vi "MBK System simulation.vi"() -> ()   [LabVIEW 2018]
uses:
  <vilib>/Analysis/3filter.llb/Filter Passband Type.ctl
  <vilib>/DAQmx/write.llb/DAQmx Write (Analog 1D DBL NChan 1Samp).vi
  <vilib>/DAQmx/read.llb/DAQmx Read (Analog 1D DBL NChan 1Samp).vi
  <vilib>/DAQmx/create/channels.llb/DAQmx Create Channel (AO-Voltage-Basic).vi
  <vilib>/DAQmx/create/channels.llb/DAQmx Create Channel (AI-Voltage-Basic).vi
  <vilib>/DAQmx/miscellaneous.llb/DAQmx Fill In Error Info.vi
  <vilib>/ptbypt/NI_PtbyPt.lvlib
  <vilib>/Analysis/NI_AALBase.lvlib
panel:
  out "Measured Acceleration":dbl(graph)
  in  "K":dbl min=0.0 max=10.0 step=0.001
  in  "Force filter Y/N":bool
  out "Desired Vel":dbl(graph)
  out "Desired acc":dbl(graph)
  in  "I_app_wall":dbl min=0.0 max=1.0 step=1e-05
  in  "I_app_transp":dbl=1e-06 min=1e-06 max=0.1 step=1e-06
  in  "B":dbl min=0.0 max=1.0 step=0.0001
  out "Velocity Meas":dbl(graph)
  in  "Vel Fil Y/N":bool
  in  "Loop Frequency":dbl
  out "Position Measured":dbl(graph)
  in  "Pos Fil Y/N":bool
  out "Force measure":dbl(graph)
  in  "stop":bool
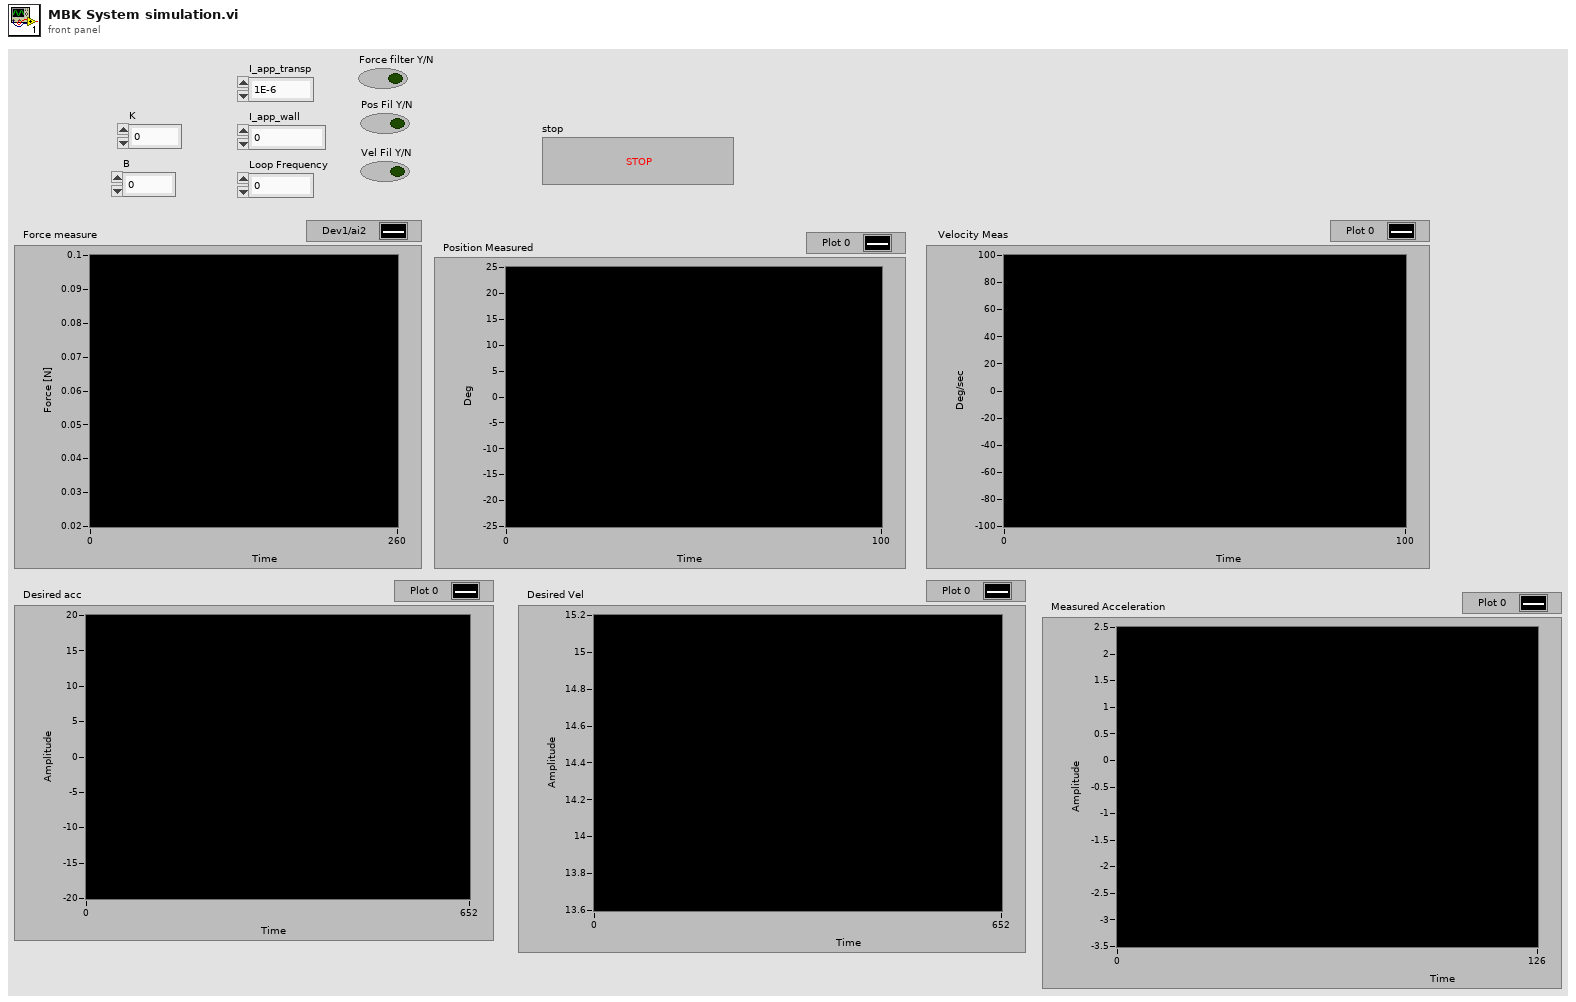
[diagram p1: front panel]
types:
  T1 = typedef "NI_AALBase.lvlib/Filter Passband Type.ctl" = enum32{"Lowpass", "Highpass", "Bandpass", "Bandstop"}
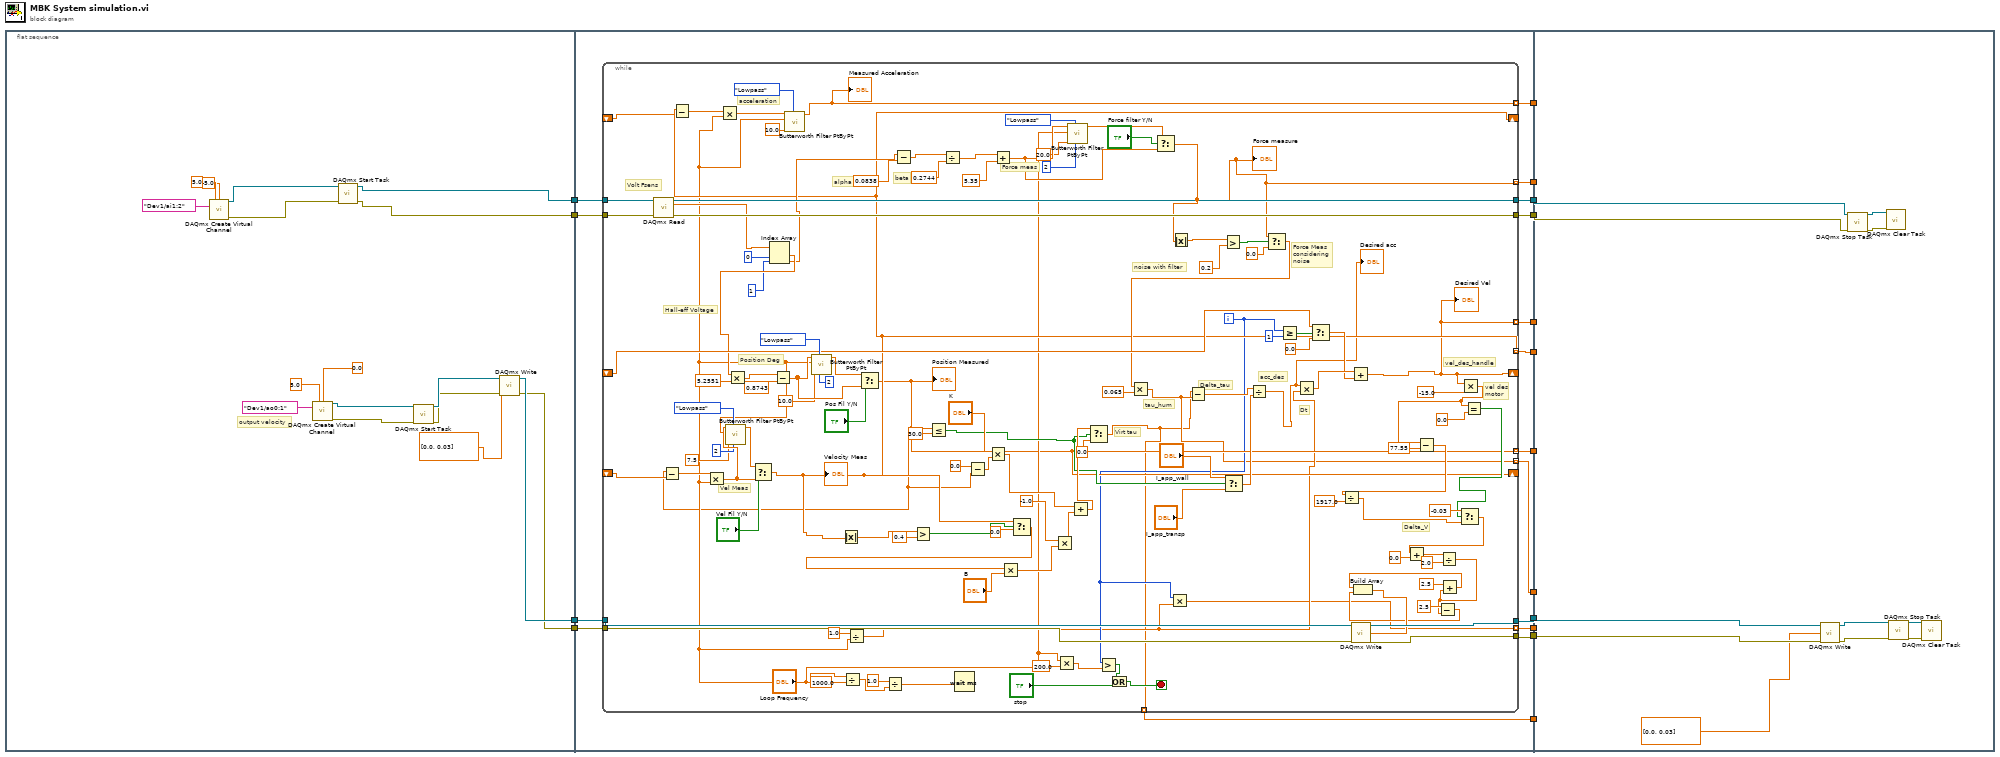
[diagram p0: block diagram]
diagram:
  n1 = flat-sequence {
    tunnel: [w30] -> w14
    tunnel: [w27] -> w12
    tunnel: [w17] -> w10
    tunnel: [w18] -> w9
    tunnel: [w49] -> w16
    tunnel: [w48] -> w15
    tunnel: w14 -> [w47]
    tunnel: [w46] -> w13
    tunnel: w12 -> [w45]
    tunnel: [w44] -> w11
    tunnel: w10 -> [w43]
    tunnel: w9 -> [w42]
    tunnel: [w41] -> w8
    tunnel: [w40] -> w7
    tunnel: [w39] -> w6
    tunnel: [w38] -> w5
    tunnel: [w37] -> w4
    tunnel: [w36] -> w3
    tunnel: [w35] -> w2
    tunnel: [w34] -> w1
    tunnel: w16 -> [w180]
    tunnel: w15 -> [w178]
    tunnel: w13 -> [w174]
    tunnel: w11 -> [w172]
    tunnel: w8 -> [_]
    tunnel: w7 -> [_]
    tunnel: w6 -> [_]
    tunnel: w5 -> [_]
    tunnel: w4 -> [_]
    tunnel: w3 -> [_]
    tunnel: w2 -> [_]
    tunnel: w1 -> [_]
    frame #0 {
      # "output velocity"
      n2 = call-poly <vilib>:"DAQmx Create Virtual Channel.vi"("maximum value"=5.0, "minimum value"=-5.0, "physical channels"=tag "Dev1/ai1:2") -> ("task out"=w24:refnum<k21>, "error out"=w23:errorcluster)  [unwired: 11 in]
      n3 = call-poly <vilib>:"DAQmx Create Virtual Channel.vi"("maximum value"=5.0, "minimum value"=0.0, "physical channels"=tag "Dev1/ao0:1") -> ("task out"=w32:refnum<k21>, "error out"=w29:errorcluster)  [unwired: 11 in]
      n4 = call <vilib>:"DAQmx Start Task.vi"("task/channels in"=w24, "error in"=w23) -> ("task out"=w18:refnum<k21>, "error out"=w17:errorcluster)  [unwired: 12 in]
      n5 = call <vilib>:"DAQmx Start Task.vi"("task/channels in"=w32, "error in"=w29) -> ("task out"=w31:refnum<k21>, "error out"=w28:errorcluster)  [unwired: 12 in]
      n6 = call-poly <vilib>:"DAQmx Write.vi"("task/channels in"=w31, "data"=dbl[] [0.0, 0.03], "error in"=w28) -> ("task out"=w30:refnum<k21>, "error out"=w27:errorcluster)  [unwired: 10 in, 1 out]
    }
    frame #1 {
      n7 = while {
        tunnel: [w169] -> w49
        tunnel: [w168] -> w48
        tunnel: w47 -> [w164]
        tunnel: [w163] -> w46
        tunnel: w45 -> [w162]
        tunnel: [w161] -> w44
        shift-right: [w59] -> _
        shift-left: _ -> [w99]
        tunnel: w43 -> [w137]
        tunnel: w42 -> [w136]
        shift-right: [w52] -> _
        shift-left: _ -> [w122]
        tunnel: [w75] -> w41 mode=indexing
        tunnel: [w74] -> w40 mode=indexing
        shift-right: [w74] -> _
        shift-left: _ -> [w73]
        tunnel: [w62] -> w39 mode=indexing
        tunnel: [w52] -> w38 mode=indexing
        tunnel: [w59] -> w37 mode=indexing
        tunnel: [w51] -> w36 mode=indexing
        tunnel: [w50] -> w35 mode=indexing
        tunnel: [w56] -> w34 mode=indexing
        i -> [w58]
        stop <- w63 stop-if-true
        # "acceleration"
        # "vel des\nmotor"
        # "Dt"
        # "Force Meas\nconsidering\nnoise"
        # "noise with filter"
        # "Force meas"
        # "Virt tau"
        # "Vel Meas"
        # "Hall-eff Voltage"
        # "Delta_tau"
        # "tau_hum"
        # "vel_des_handle"
        # "Delta_V"
        # "acc_des"
        # "Position Deg"
        # "Volt Fsens"
        # "beta"
        # "alpha"
        n8 = call-poly <vilib>:"DAQmx Read.vi"("task/channels in"=w136, "error in"=w137) -> ("task out"=w169:refnum<k21>, "data"=w138:dbl[], "error out"=w168:errorcluster)  [unwired: 11 in]
        n9 = Index Array(array=w138, index #1=0 ("index"), index #2=1 ("index")) -> (element #1=w107:dbl, element #2=w106:dbl)
        n10 = Multiply(x=w107, y=5.2551) -> (x*y=w159:dbl)
        n11 = Subtract(x=w159, y=0.8743) -> (x-y=w155:dbl)
        n12 = call <vilib>:"Butterworth Filter PtByPt.vi"("order"=2, "filter type"=Filter_Passband_Type."Lowpass", "low cutoff freq: fl"=10.0, "sampling freq: fs"="Loop Frequency", "x"=w155) -> ("Filtered x"=w156:dbl)  [unwired: 4 in, 1 out]
        n13 = Divide(x="Loop Frequency", y=1000.0) -> (x/y=w150:dbl)
        n14 = Divide(x=1.0, y="Loop Frequency") -> (x/y=w57:dbl)
        n15 = Select(t=w156, s="Pos Fil Y/N", f=w155) -> (s? t:f=w59:dbl)
        "Position Measured" <- w59
        n16 = Subtract(x=w59, y=w99) -> (x-y=w147:dbl)
        n17 = Multiply(x=w147, y="Loop Frequency") -> (x*y=w145:dbl)
        n18 = call <vilib>:"Butterworth Filter PtByPt.vi"("order"=2, "filter type"=Filter_Passband_Type."Lowpass", "low cutoff freq: fl"=7.5, "sampling freq: fs"="Loop Frequency", "x"=w145) -> ("Filtered x"=w144:dbl)  [unwired: 4 in, 1 out]
        n19 = Select(t=w144, s="Vel Fil Y/N", f=w145) -> (s? t:f=w74:dbl)
        "Velocity Meas" <- w74
        n20 = Subtract(x=w74, y=w73) -> (x-y=w72:dbl)
        n21 = Multiply(x=w72, y="Loop Frequency") -> (x*y=w71:dbl)
        n22 = call <vilib>:"Butterworth Filter PtByPt.vi"("filter type"=Filter_Passband_Type."Lowpass", "low cutoff freq: fl"=10.0, "sampling freq: fs"="Loop Frequency", "x"=w71) -> ("Filtered x"=w62:dbl)  [unwired: 5 in, 1 out]
        "Measured Acceleration" <- w62
        n23 = Absolute Value(x=w74) -> (abs(x)=w98:dbl)
        n24 = Divide(x=1.0, y=w150) -> (x/y=w135:dbl)
        n25 = Subtract(x=w106, y=0.0838) -> (x-y=w167:dbl)
        n26 = Greater?(x=w98, y=0.4) -> (0:w96:bool)
        n27 = Less Or Equal?(x=w59, y=30.0) -> (x <= y?=w77:bool)
        n28 = Divide(x=w167, y=0.2744) -> (x/y=w118:dbl)
        n29 = Wait (ms)(milliseconds to wait=w135) -> ()  [unwired: 1 out]
        n30 = Subtract(x=0.0, y=w59) -> (x-y=w88:dbl)
        n31 = Multiply(x="K", y=w88) -> (x*y=w86:dbl)
        n32 = Add(x=w118, y=5.35) -> (x+y=w116:dbl)
        n33 = Select(t=w74, s=w96, f=0.0) -> (s? t:f=w94:dbl)
        n34 = Multiply(x=w94, y="B") -> (x*y=w102:dbl)
        n35 = Multiply(x=-1.0, y=w102) -> (x*y=w90:dbl)
        n36 = Multiply(x="Loop Frequency", y=200.0) -> (x*y=w66:dbl)
        n37 = call <vilib>:"Butterworth Filter PtByPt.vi"("order"=2, "filter type"=Filter_Passband_Type."Lowpass", "low cutoff freq: fl"=20.0, "sampling freq: fs"="Loop Frequency", "x"=w116) -> ("Filtered x"=w117:dbl)  [unwired: 4 in, 1 out]
        n38 = Add(x=w86, y=w90) -> (x+y=w85:dbl)
        n39 = Select(t=w85, s=w77, f=0.0) -> (s? t:f=w50:dbl)
        n40 = Greater?(x=w58, y=w66) -> (0:w65:bool)
        n41 = Or(x=w65, y="stop") -> (x .or. y?=w63:bool)
        n42 = Select(t=w117, s="Force filter Y/N", f=w116) -> (s? t:f=w75:dbl)
        "Force measure" <- w75
        n43 = Multiply(x=w58, y=w57) -> (x*y=w56:dbl)
        n44 = Absolute Value(x=w75) -> (abs(x)=w108:dbl)
        n45 = Greater?(x=w108, y=0.2) -> (0:w60:bool)
        n46 = Select(t="I_app_wall", s=w77, f="I_app_transp") -> (s? t:f=w61:dbl)
        n47 = Select(t=w75, s=w60, f=0.0) -> (s? t:f=w109:dbl)
        n48 = Multiply(x=w109, y=0.065) -> (x*y=w51:dbl)
        n49 = Subtract(x=w50, y=w51) -> (x-y=w103:dbl)
        n50 = Divide(x=w103, y=w61) -> (x/y=w53:dbl)
        "Desired acc" <- w53
        n51 = Greater Or Equal?(x=w58, y=1) -> (x >= y?=w124:bool)
        n52 = Multiply(x=w53, y=w57) -> (x*y=w125:dbl)
        n53 = Select(t=w122, s=w124, f=0.0) -> (s? t:f=w120:dbl)
        n54 = Add(x=w125, y=w120) -> (x+y=w52:dbl)
        "Desired Vel" <- w52
        n55 = Multiply(x=w52, y=-15.0) -> (x*y=w78:dbl)
        n56 = Subtract(x=w78, y=77.55) -> (x-y=w92:dbl)
        n57 = Divide(x=w92, y=1917.0) -> (x/y=w54:dbl)
        n58 = Equal?(x=w78, y=0.0) -> (x = y?=w76:bool)
        n59 = Select(t=-0.03, s=w76, f=w54) -> (s? t:f=w55:dbl)
        n60 = Add(x=w55, y=0.0) -> (x+y=w132:dbl)
        n61 = Divide(x=w132, y=2.0) -> (x/y=w128:dbl)
        n62 = Subtract(x=2.5, y=w128) -> (x-y=w82:dbl)
        n63 = Add(x=2.5, y=w128) -> (x+y=w83:dbl)
        n64 = Build Array(w83, w82) -> (w95:dbl[])
        n65 = call-poly <vilib>:"DAQmx Write.vi"("task/channels in"=w164, "data"=w95, "error in"=w162) -> ("task out"=w163:refnum<k21>, "error out"=w161:errorcluster)  [unwired: 10 in, 1 out]
      }
    }
    frame #2 {
      n66 = call-poly <vilib>:"DAQmx Write.vi"("task/channels in"=w174, "data"=dbl[] [0.0, 0.03], "error in"=w172) -> ("task out"=w173:refnum<k21>, "error out"=w171:errorcluster)  [unwired: 10 in, 1 out]
      n67 = call <vilib>:"DAQmx Stop Task.vi"("task/channels in"=w180, "error in"=w178) -> ("task out"=w179:refnum<k21>, "error out"=w177:errorcluster)  [unwired: 12 in]
      n68 = call <vilib>:"DAQmx Clear Task.vi"("task in"=w179, "error in"=w177) -> ()  [unwired: 13 in, 1 out]
      n69 = call <vilib>:"DAQmx Stop Task.vi"("task/channels in"=w173, "error in"=w171) -> ("task out"=w176:refnum<k21>, "error out"=w175:errorcluster)  [unwired: 12 in]
      n70 = call <vilib>:"DAQmx Clear Task.vi"("task in"=w176, "error in"=w175) -> ()  [unwired: 13 in, 1 out]
    }
  }
